vi "LiFi_decoder.vi"() -> ()   [LabVIEW 2024]
uses:
  93b07758-5ef3-423c-b1f6-b3272c190e9f.vi
panel:
  out "ASCII Translation":string
  out "number":u32
  out "Reconstructed Transmission":bool[](array[boolean])
  out "Removed Redundancy Indicators":bool[](array[boolean])
  out "Array 2":i32[](array[numeric])
  out "Check TFTF":bool[](array[boolean])
  out "Singal Output":bool[](array[boolean])
  in  "Initital Sequence":bool[](array[boolean])
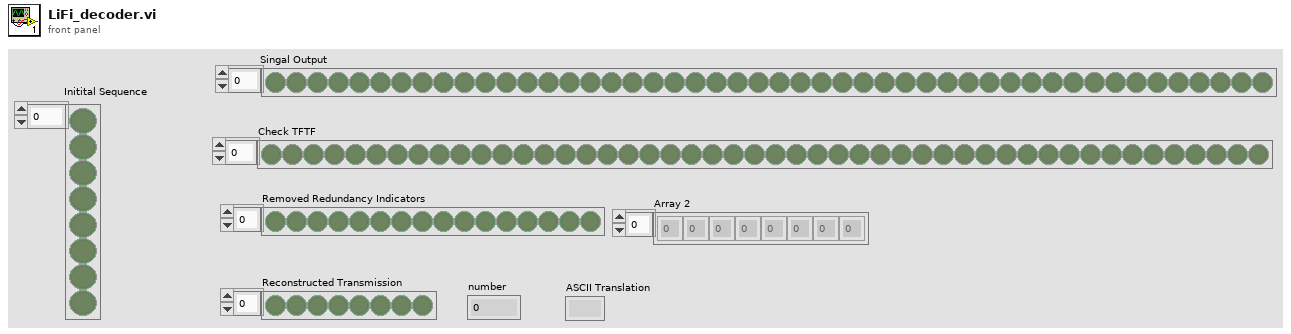
[diagram p1: front panel]
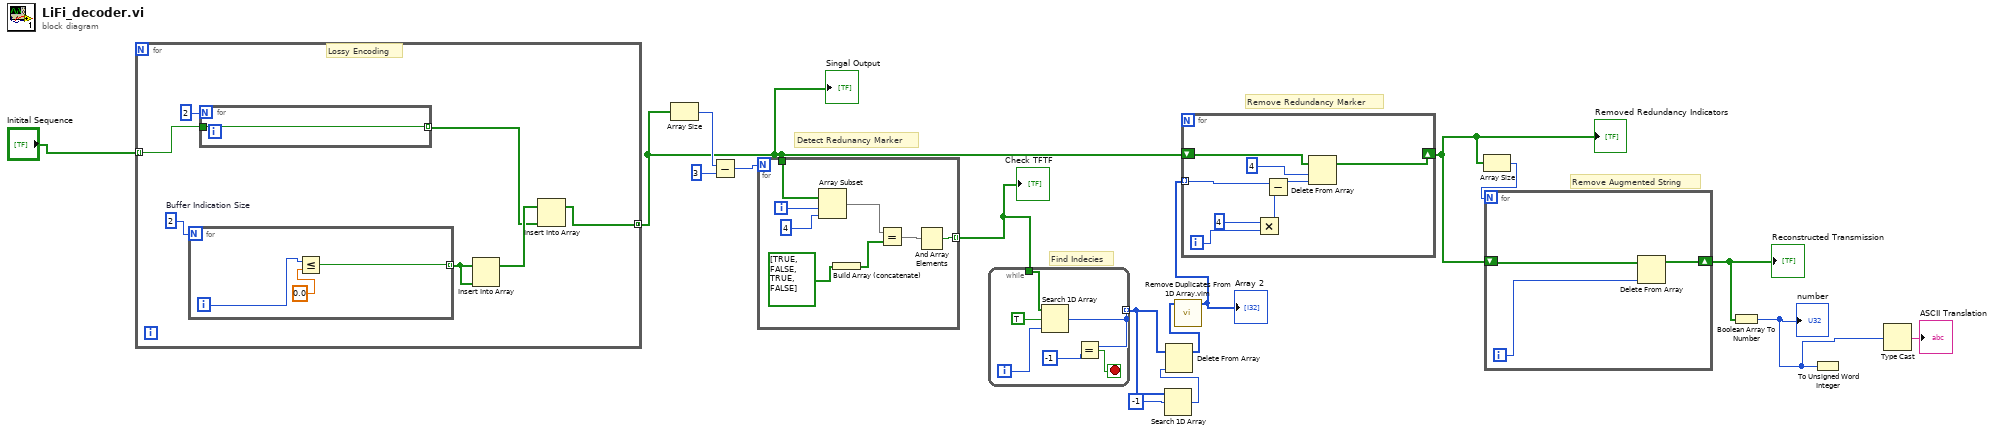
[diagram p0: block diagram]
diagram:
  # "Remove Augmented String"
  # "Remove Redundancy Marker"
  # "Find Indecies"
  # "Detect Redunancy Marker"
  n1 = for {
    tunnel: "Initital Sequence" -> [w23] mode=indexing
    tunnel: [w18] -> w6 mode=concatenating
    w22 = 2  # Buffer Indication Size
    # "Lossy Encoding"
    n2 = for {
      N: w22 -> [_]
      tunnel: [w24] -> w21 mode=indexing
      i -> [w25]
      n3 = Less Or Equal?(x=w25, y=0.0) -> (x <= y?=w24:bool)
    }
    n4 = for {
      N: 2 -> [_]
      tunnel: [w27] -> w19 mode=indexing
      tunnel: w23 -> [w27]
    }
    n5 = Insert Into Array(array=w21, new element=w21) -> (w20:bool[])  [unwired: 1 in]
    n6 = Insert Into Array(array=w20, new element=w19) -> (w18:bool[])  [unwired: 1 in]
  }
  "Singal Output" <- w6
  n7 = Array Size(array=w6) -> (size(s)=w15:i32)
  n8 = Subtract(x=w15, y=3) -> (x-y=w12:i32)
  n9 = for {
    N: w12 -> [_]
    tunnel: w6 -> [w35]
    tunnel: [w28] -> w13 mode=indexing
    i -> [w34]
    n10 = Array Subset(array=w35, index=w34, length=4) -> (w32:bool[])
    n11 = Build Array (concatenate)(bool[] [TRUE, FALSE, TRUE, FALSE] ("y")) -> (w30:bool[])
    n12 = Equal?(x=w32, y=w30) -> (x = y?=w29:bool[])
    n13 = And Array Elements(Boolean array=w29) -> (logical AND=w28:bool)
  }
  "Check TFTF" <- w13
  n14 = while {
    tunnel: w13 -> [w41]
    tunnel: [w37] -> w10 mode=indexing
    i -> [w39]
    stop <- w38 stop-if-true
    n15 = Search 1D Array(1D array=w41, element=TRUE, start index (0)=w39) -> (index of element=w37:i32)
    n16 = Equal?(x=w37, y=-1) -> (x = y?=w38:bool)
  }
  n17 = Search 1D Array(1D array=w10, element=-1 ("y")) -> (index of element=w9:i32)  [unwired: 1 in]
  n18 = Delete From Array(array=w10, index=w9) -> (array with subset deleted=w8:i32[])  [unwired: 1 in, 1 out]
  n19 = call "Remove Duplicates From 1D Array.vim"("array"=w8) -> ("array with duplicates removed"=w7:i32[])  [unwired: 10 in]
  "Array 2" <- w7
  n20 = for {
    tunnel: w7 -> [w49] mode=indexing
    shift-right: [w42] -> w5
    shift-left: w6 -> [w43]
    i -> [w47]
    n21 = Multiply(x=4, y=w47) -> (x*y=w45:i32)
    n22 = Subtract(x=w49, y=w45) -> (x-y=w48:i32)
    n23 = Delete From Array(array=w43, length=4, index=w48) -> (array with subset deleted=w42:bool[])  [unwired: 1 out]
  }
  "Removed Redundancy Indicators" <- w5
  n24 = Array Size(array=w5) -> (size(s)=w4:i32)
  n25 = for {
    N: w4 -> [_]
    shift-right: [w51] -> w3
    shift-left: w5 -> [w52]
    i -> [w50]
    n26 = Delete From Array(array=w52, index=w50) -> (array with subset deleted=w51:bool[])  [unwired: 1 in, 1 out]
  }
  "Reconstructed Transmission" <- w3
  n27 = Boolean Array To Number(Boolean array=w3) -> (number=w2:u32)
  "number" <- w2
  n28 = To Unsigned Word Integer(number=w2) -> ()  [unwired: 1 out]
  n29 = Type Cast(x=w2) -> (*(type *) &x=→"ASCII Translation":string)  [unwired: 1 in]
